vi "Build Std Wfm.vi"(8 "error in":errorcluster, 11 "Standard Wfm Config":T1={"Waveform Type"=0, "Sample Rate (Hz)"=10000000.0, "Frequency (Hz)"=10000.0, "Amplitude"=1.0, "Number of Cycles"=1, "Ramp Start"=0.0, "Ramp Stop"=1.0, "Length (s)"=0.001, "DC Value"=0.0, "Duration (s)"=0.001, "Pre Delay (s)"=0.0, "Post Delay (s)"=0.0} {"Pre Delay (s)" min=0.0 format="%#_6p"; "DC Value" format="%#_6p"; "Number of Cycles" min=1; "Duration (s)" format="%#_6p"; "Length (s)" format="%#_6p"; "Sample Rate (Hz)" min=0.0 format="%#_6p"; "Post Delay (s)" min=0.0 format="%#_6p"; "Frequency (Hz)" format="%#_6p"}) -> (0 "error out":errorcluster, 1 "Actual Duration (s)":dbl format="%#_6p", 2 "Actual Sample Size":i32, 3 "Waveform":waveform(dbl)(graph))   [LabVIEW 2025, in "TDMS Waveform Creator.lvclass"]
uses:
  TDMS Waveform Creator.lvclass
  <vilib>/Analysis/1siggen.llb/Ramp Pattern by Samples.vi
  <vilib>/Utility/error.llb/Error Cluster From Error Code.vi
  <vilib>/ErrorRing/Error Ring.xnode
  TDMS Waveform Creator.lvclass/TDMS Waveform Creator.ctl
  <vilib>/Analysis/NI_AALBase.lvlib
  TDMS Waveform Creator UI/TDMS Waveform Creator UI.lvlib
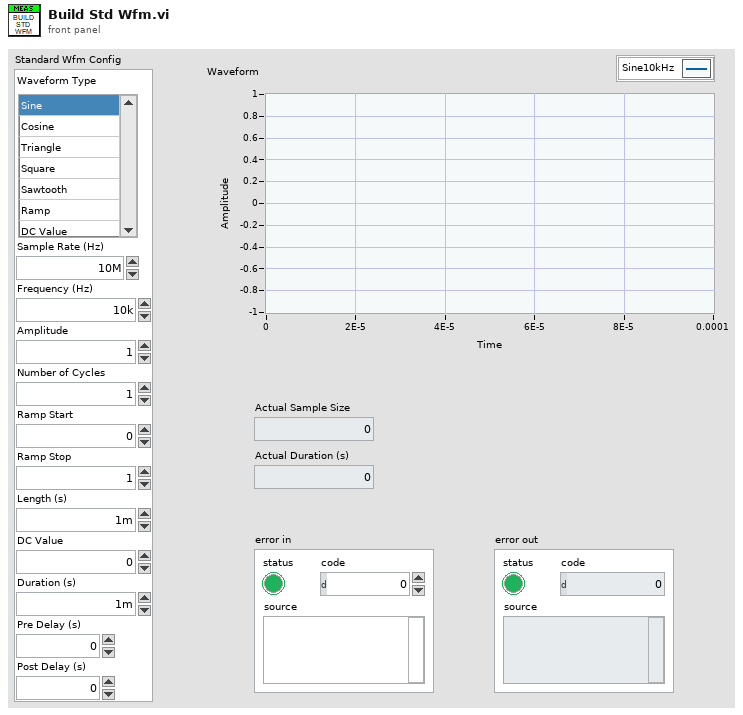
[diagram p1: front panel]
types:
  T1 = cluster{"Waveform Type":i32, "Sample Rate (Hz)":dbl, "Frequency (Hz)":dbl, "Amplitude":dbl, "Number of Cycles":u32, "Ramp Start":dbl, "Ramp Stop":dbl, "Length (s)":dbl, "DC Value":dbl, "Duration (s)":dbl, "Pre Delay (s)":dbl, "Post Delay (s)":dbl}
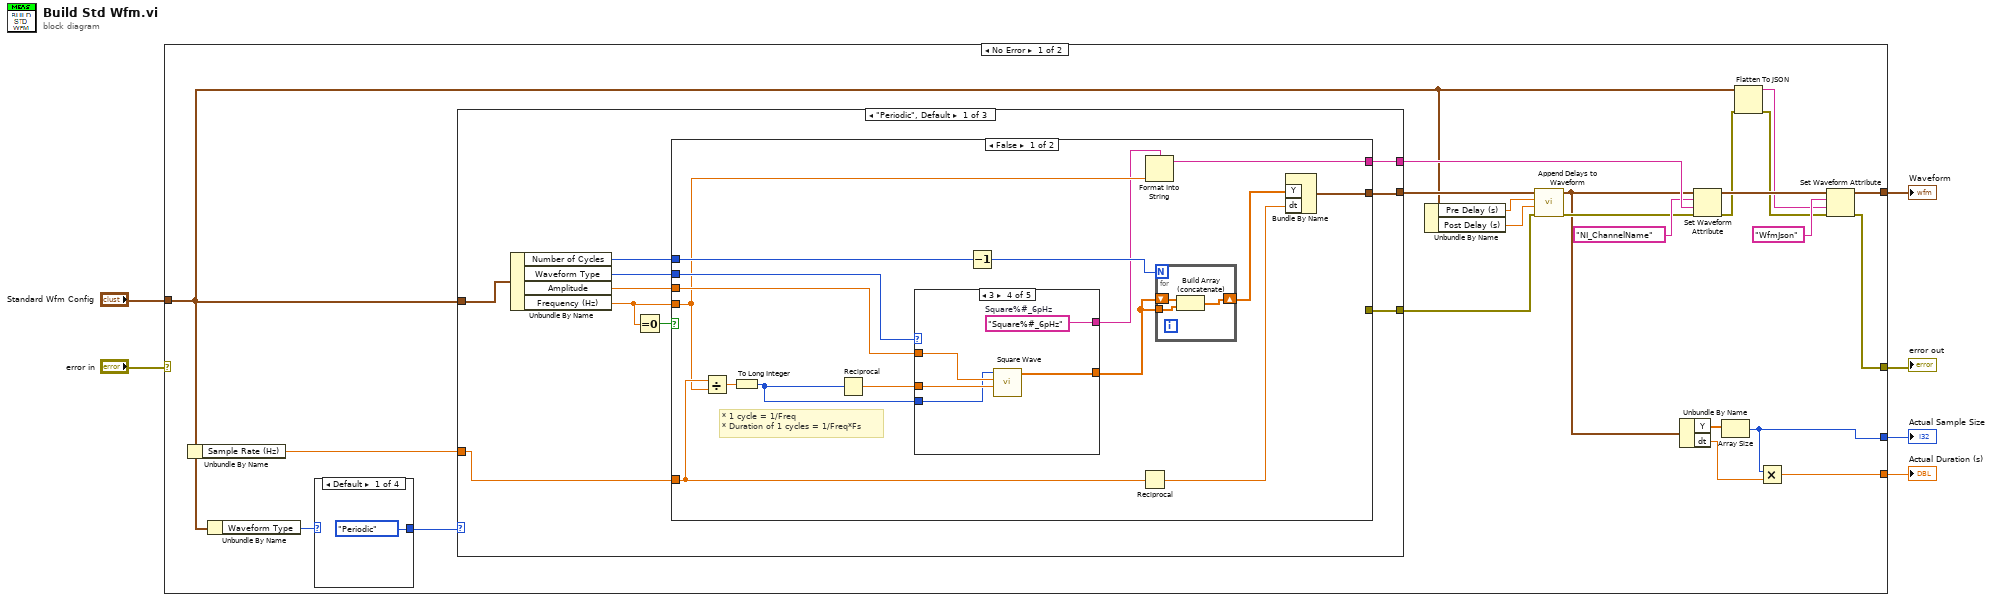
[diagram p0: block diagram]
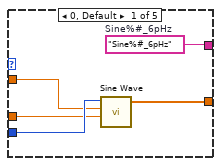
[diagram p2: hidden frame]
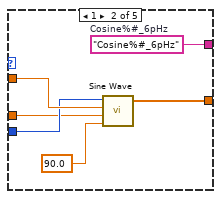
[diagram p3: hidden frame]
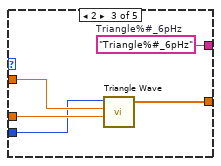
[diagram p4: hidden frame]
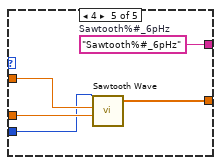
[diagram p5: hidden frame]
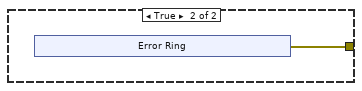
[diagram p6: hidden frame]
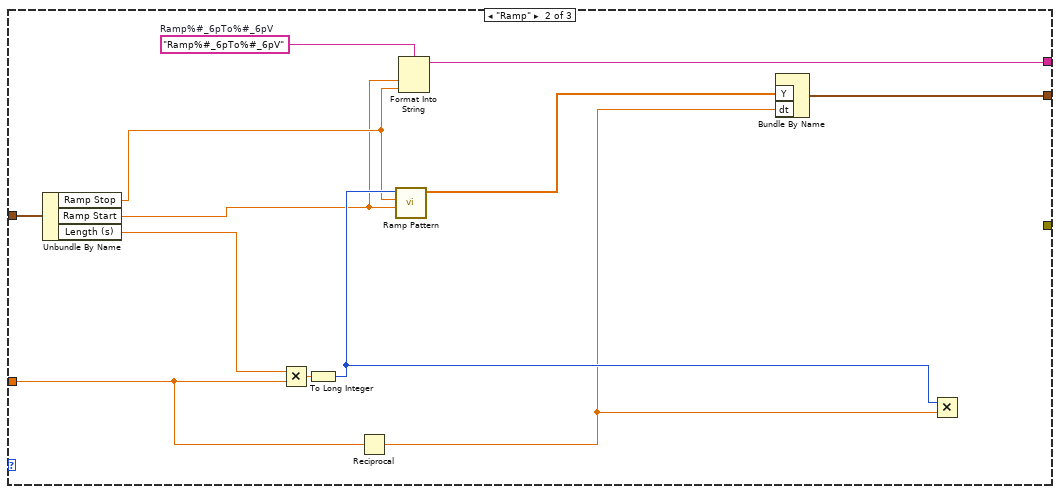
[diagram p7: hidden frame]
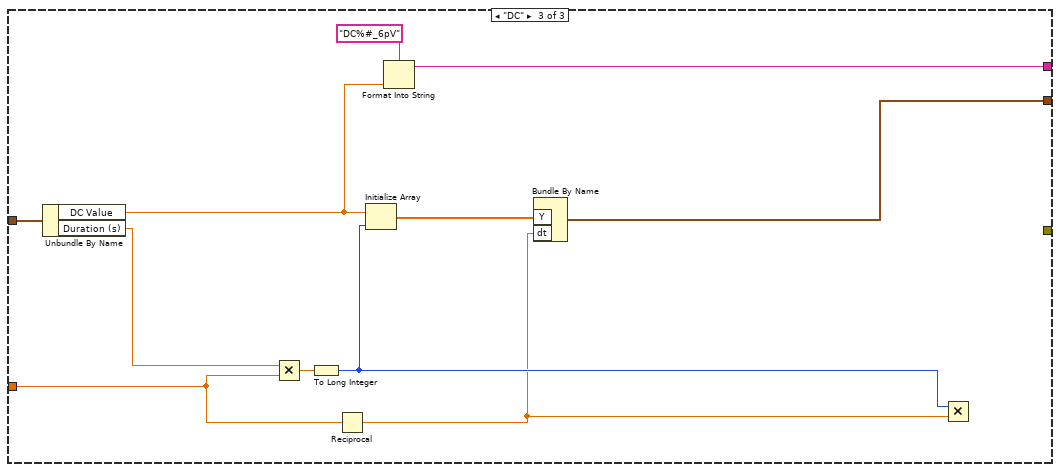
[diagram p8: hidden frame]
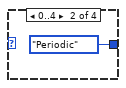
[diagram p9: hidden frame]
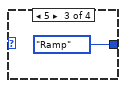
[diagram p10: hidden frame]
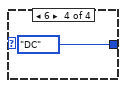
[diagram p11: hidden frame]
diagram:
  n1 = case shown="No Error" "error in" {
    selector: "error in" -> [_ w117]
    tunnel: "Standard Wfm Config" -> [w16 _]
    tunnel: [w21 _] -> w5
    tunnel: [w20 w117] -> w3
    tunnel: [w9 _] -> w2
    tunnel: [w8 _] -> w1
    frame No Error {
      n2 = Unbundle By Name(w16) -> ("Sample Rate (Hz)"=w27:dbl)
      n3 = Unbundle By Name(w16) -> ("Waveform Type"=w29:i32)
      n4 = case shown="Default" w29 {
        tunnel: [enum32{"Periodic", "Ramp", "DC"}."Periodic" ("Value (Signaling)") enum32{"Periodic", "Ramp", "DC"}."Periodic" ("Value (Signaling)") enum32{"Periodic", "Ramp", "DC"}."Ramp" ("Value (Signaling)") enum32{"Periodic", "Ramp", "DC"}."DC" ("Value (Signaling)")] -> w28
        frame Default {
        }
        frame 0..4 {
        }
        frame 5 {
        }
        frame 6 {
        }
      }
      n5 = case shown="\"Periodic\", Default" w28 {
        tunnel: w27 -> [w37 w100 w102]
        tunnel: [w38 w96 w107] -> w24
        tunnel: [w39 w98 w106] -> w19
        tunnel: w16 -> [w33 w93 w105]
        tunnel: [w30 _ _] -> w18
        frame "Periodic", Default {
          n6 = Unbundle By Name(w33) -> ("Number of Cycles"=w36:u32, "Waveform Type"=w34:i32, "Amplitude"=w35:dbl, "Frequency (Hz)"=w32:dbl)
          n7 = Equal To 0?(x=w32) -> (x = 0?=w31:bool)
          n8 = case shown="False" w31 {
            tunnel: [w54 _] -> w39
            tunnel: [w53 _] -> w38
            tunnel: w37 -> [w50 _]
            tunnel: w36 -> [w46 _]
            tunnel: w35 -> [w43 _]
            tunnel: w34 -> [w42 _]
            tunnel: w32 -> [w41 _]
            tunnel: [_ w84] -> w30
            frame False {
              # "* 1 cycle = 1/Freq\n* Duration of 1 cycles = 1/Freq*Fs"
              n9 = Divide(x=w50, y=w41) -> (x/y=w51:dbl)
              n10 = To Long Integer(number=w51) -> (32bit integer=w44:i32)
              n11 = Reciprocal(x=w44) -> (1/x=w45:dbl)
              n12 = case shown="3" w42 {
                tunnel: w43 -> [w57 w65 w70 w75 w80]
                tunnel: w44 -> [w59 w64 w68 w73 w78]
                tunnel: w45 -> [w56 w63 w69 w74 w79]
                tunnel: [w58 w61 w67 w72 w77] -> w49
                tunnel: [w55 w60 w66 w71 w76] -> w40
                frame 0, Default {
                  w55 = "Sine%#_6pHz"  # Sine%#_6pHz
                  n13 = call <vilib>:"Sine Wave.vi"("samples"=w59, "amplitude"=w57, "frequency"=w56) -> ("sine wave"=w58:dbl[])  [unwired: 2 in, 2 out]
                }
                frame 1 {
                  w60 = "Cosine%#_6pHz"  # Cosine%#_6pHz
                  n14 = call <vilib>:"Sine Wave.vi"("samples"=w64, "amplitude"=w65, "frequency"=w63, "phase in"=90.0) -> ("sine wave"=w61:dbl[])  [unwired: 1 in, 2 out]
                }
                frame 2 {
                  w66 = "Triangle%#_6pHz"  # Triangle%#_6pHz
                  n15 = call <vilib>:"Triangle Wave.vi"("samples"=w68, "amplitude"=w70, "frequency"=w69) -> ("triangle wave"=w67:dbl[])  [unwired: 2 in, 2 out]
                }
                frame 3 {
                  w71 = "Square%#_6pHz"  # Square%#_6pHz
                  n16 = call <vilib>:"Square Wave.vi"("samples"=w73, "amplitude"=w75, "frequency"=w74) -> ("square wave"=w72:dbl[])  [unwired: 3 in, 2 out]
                }
                frame 4 {
                  w76 = "Sawtooth%#_6pHz"  # Sawtooth%#_6pHz
                  n17 = call <vilib>:"Sawtooth Wave.vi"("samples"=w78, "amplitude"=w80, "frequency"=w79) -> ("sawtooth wave"=w77:dbl[])  [unwired: 2 in, 2 out]
                }
              }
              n18 = Decrement(x=w46) -> (x-1=w48:u32)
              n19 = Reciprocal(x=w50) -> (1/x=w52:dbl)
              n20 = Format Into String(format string=w40, w41) -> (resulting string=w53:string)  [unwired: 2 in, 1 out]
              n21 = for {
                N: w48 -> [_]
                shift-right: [w82] -> w47
                shift-left: w49 -> [w83]
                tunnel: w49 -> [w81]
                n22 = Build Array (concatenate)(w83, w81) -> (w82:dbl[])
              }
              n23 = Bundle By Name("Y"=w47, "dt"=w52) -> (w54:waveform(dbl))  [unwired: 1 in]
            }
            frame True {
              n24 = xnode "Error Ring"() -> ("error out"=w84:errorcluster)
            }
          }
        }
        frame "Ramp" {
          w97 = "Ramp%#_6pTo%#_6pV"  # Ramp%#_6pTo%#_6pV
          n25 = Unbundle By Name(w93) -> ("Ramp Stop"=w92:dbl, "Ramp Start"=w91:dbl, "Length (s)"=w90:dbl)
          n26 = Multiply(x=w90, y=w100) -> (x*y=w101:dbl)
          n27 = To Long Integer(number=w101) -> (32bit integer=w95:i32)
          n28 = Reciprocal(x=w100) -> (1/x=w94:dbl)
          n29 = call-poly <vilib>:"Ramp Pattern.vi"("start"=w91, "end"=w92, "samples"=w95) -> ("Ramp Pattern"=w99:dbl[])  [unwired: 7 in, 1 out]
          n30 = Format Into String(format string=w97, w91, w92) -> (resulting string=w96:string)  [unwired: 2 in, 1 out]
          n31 = Bundle By Name("Y"=w99, "dt"=w94) -> (w98:waveform(dbl))  [unwired: 1 in]
          n32 = Multiply(x=w95, y=w94) -> ()  [unwired: 1 out]
        }
        frame "DC" {
          n33 = Unbundle By Name(w105) -> ("DC Value"=w103:dbl, "Duration (s)"=w104:dbl)
          n34 = Multiply(x=w104, y=w102) -> (x*y=w112:dbl)
          n35 = To Long Integer(number=w112) -> (32bit integer=w110:i32)
          n36 = Reciprocal(x=w102) -> (1/x=w109:dbl)
          n37 = Initialize Array(w103, w110) -> (w111:dbl[])
          n38 = Format Into String(format string="DC%#_6pV", w103) -> (resulting string=w107:string)  [unwired: 2 in, 1 out]
          n39 = Bundle By Name("Y"=w111, "dt"=w109) -> (w106:waveform(dbl))  [unwired: 1 in]
          n40 = Multiply(x=w110, y=w109) -> ()  [unwired: 1 out]
        }
      }
      n41 = Unbundle By Name(w16) -> ("Pre Delay (s)"=w15:dbl, "Post Delay (s)"=w14:dbl)
      n42 = call "Append Delays to Waveform.vi"("error in (no error)"=w18, "Post Delay (s)"=w14, "Pre Delay (s)"=w15, "Input Waveform"=w19) -> ("error out"=w17:errorcluster, "Output Waveform"=w7:waveform(dbl))  [unwired: 6 in]
      n43 = Unbundle By Name(w7) -> ("Y"=w10:dbl[], "dt"=w11:dbl)
      n44 = Set Waveform Attribute(4:w17, 5:w24, 6:"NI_ChannelName" ("name"), 7:w7) -> (0:w13:errorcluster, 3:w26:waveform(dbl))  [unwired: 1 out]
      n45 = Array Size(array=w10) -> (size(s)=w9:i32)
      n46 = Flatten To JSON(anything=w16, error in (no error)=w13) -> (JSON string=w22:string, 11:w12:errorcluster)  [unwired: 1 in]
      n47 = Multiply(x=w9, y=w11) -> (x*y=w8:dbl)
      n48 = Set Waveform Attribute(4:w12, 5:w22, 6:"WfmJson" ("name"), 7:w26) -> (0:w20:errorcluster, 3:w21:waveform(dbl))  [unwired: 1 out]
    }
    frame Error {
    }
  }
  "Actual Duration (s)" <- w1
  "Actual Sample Size" <- w2
  "Waveform" <- w5
  "error out" <- w3
